vi "zSpecJSON.vi"(8 "Error in (no error)":errorcluster, 11 "Application ref in":refnum<vi>) -> (0 "Error out":errorcluster, 2 "JSON string":string, 3 "Application ref out":refnum<vi>)   [LabVIEW 2021]
uses:
  <userlib>/Nanonis Prog Interface V5/Nanonis Prog Interface.lvlib
panel:
  out "Retract condition":enum16{">", "<"}(ring) caption="Auto retract condition"
  in  "zSpec":T1={"Parameters"=[], "Number of points"=0, "Fixed parameters"=[], "Backward sweep"=FALSE, "Z offset (m)"=nan, "Z distance (m)"=nan, "Retract delay (s)"=nan, "Channels"=[], "Time between forward and backward sweep (s)"=0.0, "Lock-In run during measurement"=FALSE, "Reset Z at the end of the sweep"=FALSE, "Record final Z position at the end of the sweep"=FALSE, "Multiple sweeps configuration"={"Number of  Sweeps"=0, "Save all"=FALSE}, "Sweep Timing"={"Max. slew rate (m/s)"=0.0, "Settling time (s)"=0.0, "Integration time (s)"=0.0}, "End of Sweep"={"End settling time (s)"=0.0, "Z control time (s)"=0.0}, "Initialization"={"Z averaging time (s)"=0.0, "Initial settling time (s)"=0.0}, "RetractCondition"=""} {"Initialization"."Initial settling time (s)" step=0.0001 format="%.3p"; "Initialization"."Z averaging time (s)" min=0 max=10 step=0.0001 format="%.3p"; "End of Sweep"."Z control time (s)" min=0 max=10 step=0.0001 format="%.3p"; "End of Sweep"."End settling time (s)" step=0.0001 format="%.3p"; "Sweep Timing"."Integration time (s)" min=0 max=20 step=0.0001 format="%.3p"; "Sweep Timing"."Settling time (s)" step=0.0001 format="%.3p"; "Sweep Timing"."Max. slew rate (m/s)" format="%.3p"; "Time between forward and backward sweep (s)" format="%#_4p"; "Retract delay (s)" format="%.3p"; "Z distance (m)" format="%.3p"; "Z offset (m)" format="%.3p"}
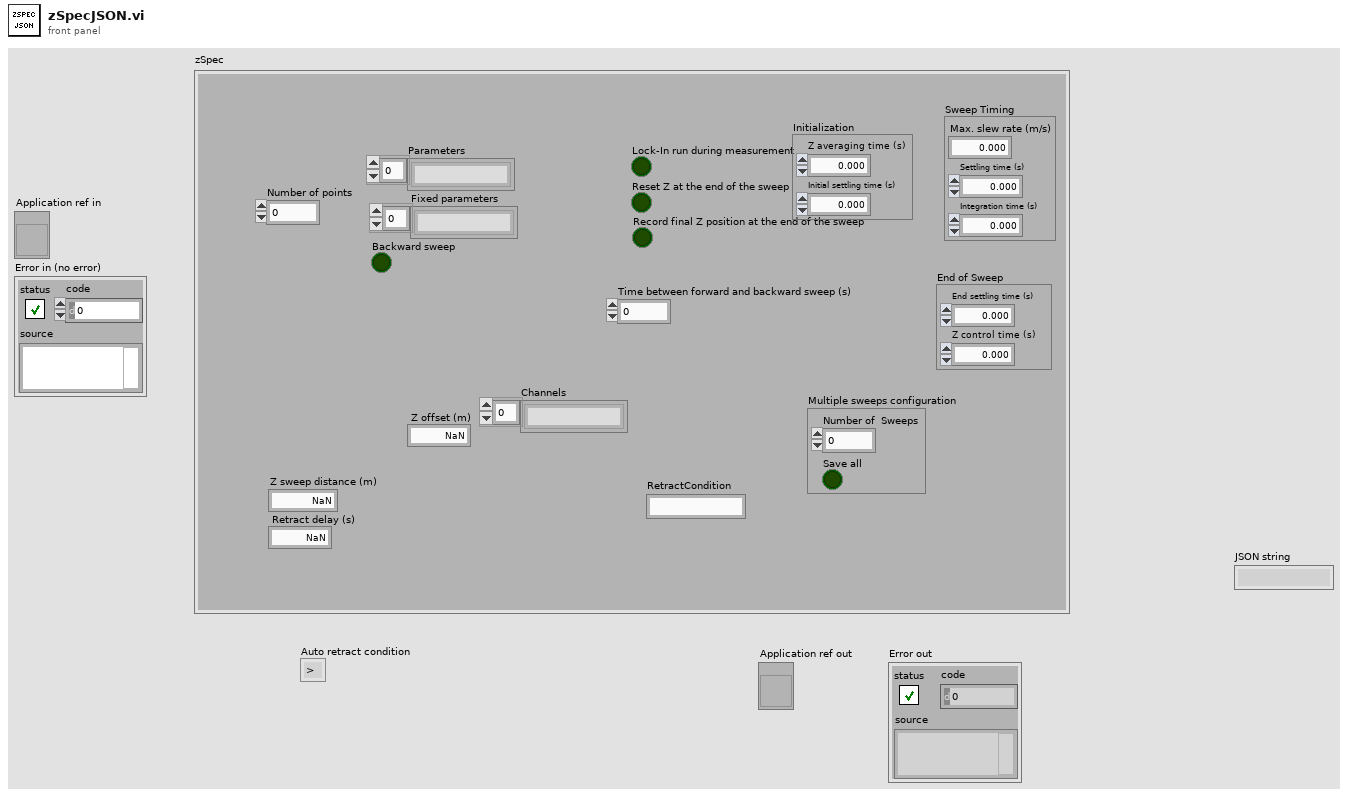
[diagram p1: front panel]
types:
  T1 = cluster{"Parameters":string[], "Number of points":i32, "Fixed parameters":string[], "Backward sweep":bool, "Z offset (m)":sgl, "Z distance (m)":sgl, "Retract delay (s)":sgl, "Channels":string[], "Time between forward and backward sweep (s)":sgl, "Lock-In run during measurement":bool, "Reset Z at the end of the sweep":bool, "Record final Z position at the end of the sweep":bool, "Multiple sweeps configuration":cluster{"Number of  Sweeps":i32, "Save all":bool}, "Sweep Timing":cluster{"Max. slew rate (m/s)":sgl, "Settling time (s)":sgl, "Integration time (s)":sgl}, "End of Sweep":cluster{"End settling time (s)":sgl, "Z control time (s)":sgl}, "Initialization":cluster{"Z averaging time (s)":sgl, "Initial settling time (s)":sgl}, "RetractCondition":string}
  T2 = cluster{"Number of  Sweeps":i32, "Save all":bool}
  T3 = cluster{"Z averaging time (s)":sgl, "Initial settling time (s)":sgl}
  T4 = cluster{"Max. slew rate (m/s)":sgl, "Settling time (s)":sgl, "Integration time (s)":sgl}
  T5 = cluster{"End settling time (s)":sgl, "Z control time (s)":sgl}
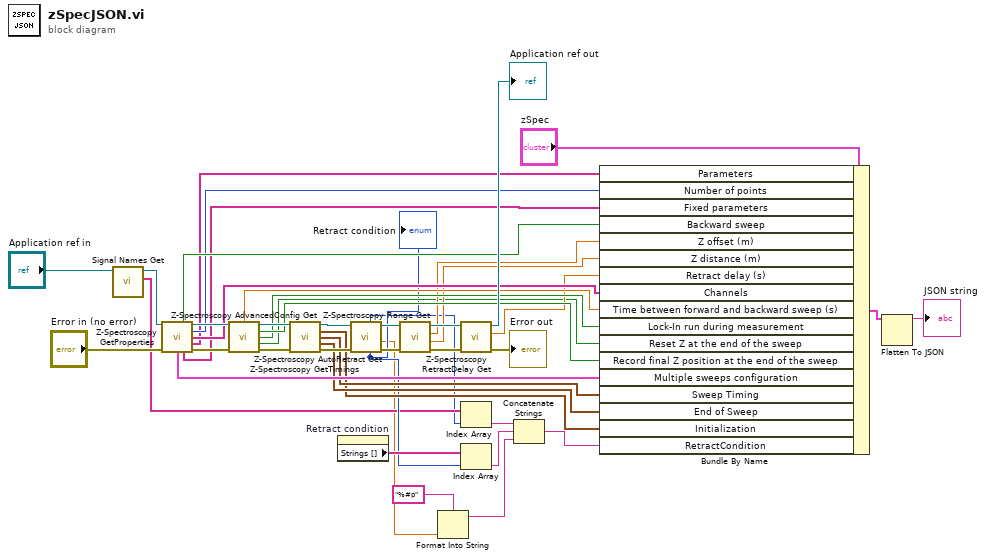
[diagram p0: block diagram]
diagram:
  n1 = call <userlib>:"Signal Names Get.vi"("Application ref in"="Application ref in") -> ("Signals Names"=w8:string[], "Application ref out"=w9:refnum<vi>)  [unwired: 6 in, 1 out]
  n2 = call <userlib>:"Z-Spectroscopy GetProperties.vi"("Application ref in"=w9, "error in (no error)"="Error in (no error)") -> ("Backward sweep"=w29:bool, "Application ref out"=w43:refnum<vi>, "Number of points"=w28:i32, "Channels"=w27:string[], "Parameters"=w26:string[], "Multiple sweeps configuration"=w16:T2, "Fixed parameters"=w25:string[], "error out"=w37:errorcluster)  [unwired: 6 in]
  n3 = call <userlib>:"Z-Spectroscopy AdvancedConfig Get.vi"("Application ref in"=w43, "error in (no error)"=w37) -> ("Time between forward and backward sweep (s)"=w24:sgl, "Application ref out"=w42:refnum<vi>, "Record final Z position at the end of the sweep"=w23:bool, "Lock-In run during measurement"=w22:bool, "Reset Z at the end of the sweep"=w18:bool, "error out"=w36:errorcluster)  [unwired: 8 in]
  n4 = call <userlib>:"Z-Spectroscopy GetTimings.vi"("Application ref in"=w42, "Error in (no error)"=w36) -> ("Application ref out"=w41:refnum<vi>, "Initialization"=w13:T3, "Sweep Timing"=w15:T4, "End of Sweep"=w14:T5, "Error out"=w35:errorcluster)  [unwired: 9 in]
  n5 = property on="Retract condition" class="Enum (strict)"() -> ("Strings []"=w12:string[])  [unwired: 2 in, 2 out]
  n6 = call <userlib>:"Z-Spectroscopy AutoRetract Get.vi"("error in (no error)"=w35, "Application ref in"=w41) -> ("error out"=w34:errorcluster, "Threshold"=w2:sgl, "Application ref out"=w40:refnum<vi>, "Retract condition"=w11:enum16{">", "<"}, "Signal Index"=w7:i32)  [unwired: 4 in, 1 out]
  "Retract condition" <- w11
  n7 = call <userlib>:"Z-Spectroscopy Range Get.vi"("error in (no error)"=w34, "Application ref in"=w40) -> ("error out"=w33:errorcluster, "Z distance (m)"=w20:sgl, "Z offset (m)"=w21:sgl, "Application ref out"=w39:refnum<vi>)  [unwired: 5 in]
  n8 = Format Into String(format string="%#p", w2) -> (resulting string=w3:string)  [unwired: 2 in, 1 out]
  n9 = call <userlib>:"Z-Spectroscopy RetractDelay Get.vi"("error in (no error)"=w33, "Application ref in"=w39) -> ("error out"=→"Error out":errorcluster, "Retract delay (s)"=w19:sgl, "Application ref out"=→"Application ref out":refnum<vi>)  [unwired: 7 in]
  n10 = Index Array(array=w8, index=w7) -> (element=w6:string)
  n11 = Index Array(array=w12, index=w11) -> (element=w4:string)
  n12 = Concatenate Strings(w6, w4, w3) -> (w5:string)
  n13 = Bundle By Name(cluster="zSpec", "Parameters"=w26, "Number of points"=w28, "Fixed parameters"=w25, "Backward sweep"=w29, "Z offset (m)"=w21, "Z distance (m)"=w20, "Retract delay (s)"=w19, "Channels"=w27, "Time between forward and backward sweep (s)"=w24, "Lock-In run during measurement"=w22, "Reset Z at the end of the sweep"=w18, "Record final Z position at the end of the sweep"=w23, "Multiple sweeps configuration"=w16, "Sweep Timing"=w15, "End of Sweep"=w14, "Initialization"=w13, "RetractCondition"=w5) -> (w17:T1)
  n14 = Flatten To JSON(anything=w17) -> (JSON string=→"JSON string":string)  [unwired: 2 in, 1 out]
